vi "S4GUI.vi"(7 "Tab ObsEng":enum32{"Obs", "CCD modes", "Guider", "Eng"}(tab)) -> ()   [LabVIEW 2018] (continued)
        n5074 = call-dynamic "Write Focus.vi"("error in (no error)"=w12180, "GSdevice.lvclass"=w12182, "GSserver in"=w12181) -> ("error out"=w12177:errorcluster, "GSserver out"=w12179:refnum<class "GSserver.lvclass">)  [unwired: 7 in]
        n5075 = call-dynamic "Write GSserver.lvclass.vi"("error in (no error)"=w12177, "GSserver.lvclass"=w12179, "S4GUI in"=w12178) -> ("error out"=w12176:errorcluster, "S4GUI out"=w12175:refnum<class "S4GUI.lvclass">)  [unwired: 7 in]
      }
      event "GFOC_set": Value Change {
        n5076 = event-data() -> ()  [unwired: 1 in, 4 out]
        n5077 = call "Read Instrument.lvclass.vi"("error in (no error)"=w12207, "S4ACS_GUI in"=w12208) -> ("error out"=w12205:errorcluster, "Instrument.lvclass"=w12206:refnum<class "Instrument.lvclass">, "S4ACS_GUI out"=w12193:refnum<class "S4GUI.lvclass">)  [unwired: 7 in]
        n5078 = call "Read GFOC.vi"("error in (no error)"=w12205, "Instrument in"=w12206) -> ("error out"=w12202:errorcluster, "Opt_Continuous.lvclass"=w12204:refnum<class "Opt_Continuous.lvclass">, "Instrument out"=w12196:refnum<class "Instrument.lvclass">)  [unwired: 7 in]
        n5079 = call-dynamic "Read State Machine.vi"("error in (no error)"=w12202, "Device in"=w12204) -> ("error out"=w12201:errorcluster, "State Machine.lvclass"=w12190:refnum<class "State Machine.lvclass">, "Device out"=w12198:refnum<class "Opt_Continuous.lvclass">)  [unwired: 7 in]
        n5080 = call "Next State.vi"("error in (no error)"=w12201, "New_State"=1, "State Machine in"=w12190) -> ("error out"=w12200:errorcluster, "State Machine out"=w12199:refnum<class "State Machine.lvclass">)  [unwired: 7 in]
        n5081 = call-dynamic "Write State Machine.vi"("error in (no error)"=w12200, "State Machine.lvclass"=w12199, "Device in"=w12198) -> ("error out"=w12195:errorcluster, "Device out"=w12197:refnum<class "Opt_Continuous.lvclass">)  [unwired: 7 in]
        n5082 = call "Write GFOC.vi"("error in (no error)"=w12195, "Opt_Continuous.lvclass"=w12197, "Instrument in"=w12196) -> ("error out"=w12192:errorcluster, "Instrument out"=w12194:refnum<class "Instrument.lvclass">)  [unwired: 7 in]
        n5083 = call "Write Instrument.lvclass.vi"("error in (no error)"=w12192, "Instrument.lvclass"=w12194, "S4ACS_GUI in"=w12193) -> ("error out"=w12191:errorcluster, "S4ACS_GUI out"=w12189:refnum<class "S4GUI.lvclass">)  [unwired: 7 in]
      }
      event "GFOC_set 2": Value Change {
        n5084 = event-data() -> ()  [unwired: 1 in, 4 out]
        n5085 = call-dynamic "Read GSserver.lvclass.vi"("error in (no error)"=w12227, "S4GUI in"=w12228) -> ("error out"=w12225:errorcluster, "GSserver.lvclass"=w12226:refnum<class "GSserver.lvclass">, "S4GUI out"=w12213:refnum<class "S4GUI.lvclass">)  [unwired: 7 in]
        n5086 = call-dynamic "Read Focus.vi"("error in (no error)"=w12225, "GSserver in"=w12226) -> ("error out"=w12222:errorcluster, "GSdevice.lvclass"=w12224:refnum<class "GSdevice.lvclass">, "GSserver out"=w12216:refnum<class "GSserver.lvclass">)  [unwired: 7 in]
        n5087 = call-dynamic "Read State Machine.vi"("error in (no error)"=w12222, "Device in"=w12224) -> ("error out"=w12221:errorcluster, "State Machine.lvclass"=w12210:refnum<class "State Machine.lvclass">, "Device out"=w12218:refnum<class "GSdevice.lvclass">)  [unwired: 7 in]
        n5088 = call "Next State.vi"("error in (no error)"=w12221, "New_State"=10, "State Machine in"=w12210) -> ("error out"=w12220:errorcluster, "State Machine out"=w12219:refnum<class "State Machine.lvclass">)  [unwired: 7 in]
        n5089 = call-dynamic "Write State Machine.vi"("error in (no error)"=w12220, "State Machine.lvclass"=w12219, "Device in"=w12218) -> ("error out"=w12215:errorcluster, "Device out"=w12217:refnum<class "GSdevice.lvclass">)  [unwired: 7 in]
        n5090 = call-dynamic "Write Focus.vi"("error in (no error)"=w12215, "GSdevice.lvclass"=w12217, "GSserver in"=w12216) -> ("error out"=w12212:errorcluster, "GSserver out"=w12214:refnum<class "GSserver.lvclass">)  [unwired: 7 in]
        n5091 = call-dynamic "Write GSserver.lvclass.vi"("error in (no error)"=w12212, "GSserver.lvclass"=w12214, "S4GUI in"=w12213) -> ("error out"=w12211:errorcluster, "S4GUI out"=w12209:refnum<class "S4GUI.lvclass">)  [unwired: 7 in]
      }
      event "GFOC_stop", "GFOC_stop 2": Value Change {
        n5092 = event-data() -> ()  [unwired: 1 in, 4 out]
        n5093 = call "Read Instrument.lvclass.vi"("error in (no error)"=w12247, "S4ACS_GUI in"=w12248) -> ("error out"=w12245:errorcluster, "Instrument.lvclass"=w12246:refnum<class "Instrument.lvclass">, "S4ACS_GUI out"=w12232:refnum<class "S4GUI.lvclass">)  [unwired: 7 in]
        n5094 = call "Read GFOC.vi"("error in (no error)"=w12245, "Instrument in"=w12246) -> ("error out"=w12241:errorcluster, "Opt_Continuous.lvclass"=w12244:refnum<class "Opt_Continuous.lvclass">, "Instrument out"=w12235:refnum<class "Instrument.lvclass">)  [unwired: 7 in]
        n5095 = call-dynamic "Read State Machine.vi"("error in (no error)"=w12241, "Device in"=w12244) -> ("error out"=w12240:errorcluster, "State Machine.lvclass"=w12243:refnum<class "State Machine.lvclass">, "Device out"=w12237:refnum<class "Opt_Continuous.lvclass">)  [unwired: 7 in]
        n5096 = call "Next State.vi"("error in (no error)"=w12240, "New_State"=10, "State Machine in"=w12243) -> ("error out"=w12239:errorcluster, "State Machine out"=w12238:refnum<class "State Machine.lvclass">)  [unwired: 7 in]
        n5097 = call-dynamic "Write State Machine.vi"("error in (no error)"=w12239, "State Machine.lvclass"=w12238, "Device in"=w12237) -> ("error out"=w12234:errorcluster, "Device out"=w12236:refnum<class "Opt_Continuous.lvclass">)  [unwired: 7 in]
        n5098 = call "Write GFOC.vi"("error in (no error)"=w12234, "Opt_Continuous.lvclass"=w12236, "Instrument in"=w12235) -> ("error out"=w12231:errorcluster, "Instrument out"=w12233:refnum<class "Instrument.lvclass">)  [unwired: 7 in]
        n5099 = call "Write Instrument.lvclass.vi"("error in (no error)"=w12231, "Instrument.lvclass"=w12233, "S4ACS_GUI in"=w12232) -> ("error out"=w12230:errorcluster, "S4ACS_GUI out"=w12229:refnum<class "S4GUI.lvclass">)  [unwired: 7 in]
      }
      event "GFOC_init": Value Change {
        n5100 = event-data() -> ()  [unwired: 1 in, 4 out]
        n5101 = call "Read Instrument.lvclass.vi"("error in (no error)"=w12267, "S4ACS_GUI in"=w12268) -> ("error out"=w12265:errorcluster, "Instrument.lvclass"=w12266:refnum<class "Instrument.lvclass">, "S4ACS_GUI out"=w12252:refnum<class "S4GUI.lvclass">)  [unwired: 7 in]
        n5102 = call "Read GFOC.vi"("error in (no error)"=w12265, "Instrument in"=w12266) -> ("error out"=w12261:errorcluster, "Opt_Continuous.lvclass"=w12264:refnum<class "Opt_Continuous.lvclass">, "Instrument out"=w12255:refnum<class "Instrument.lvclass">)  [unwired: 7 in]
        n5103 = call-dynamic "Read State Machine.vi"("error in (no error)"=w12261, "Device in"=w12264) -> ("error out"=w12260:errorcluster, "State Machine.lvclass"=w12263:refnum<class "State Machine.lvclass">, "Device out"=w12257:refnum<class "Opt_Continuous.lvclass">)  [unwired: 7 in]
        n5104 = call "Next State.vi"("error in (no error)"=w12260, "New_State"=30, "State Machine in"=w12263) -> ("error out"=w12259:errorcluster, "State Machine out"=w12258:refnum<class "State Machine.lvclass">)  [unwired: 7 in]
        n5105 = call-dynamic "Write State Machine.vi"("error in (no error)"=w12259, "State Machine.lvclass"=w12258, "Device in"=w12257) -> ("error out"=w12254:errorcluster, "Device out"=w12256:refnum<class "Opt_Continuous.lvclass">)  [unwired: 7 in]
        n5106 = call "Write GFOC.vi"("error in (no error)"=w12254, "Opt_Continuous.lvclass"=w12256, "Instrument in"=w12255) -> ("error out"=w12251:errorcluster, "Instrument out"=w12253:refnum<class "Instrument.lvclass">)  [unwired: 7 in]
        n5107 = call "Write Instrument.lvclass.vi"("error in (no error)"=w12251, "Instrument.lvclass"=w12253, "S4ACS_GUI in"=w12252) -> ("error out"=w12250:errorcluster, "S4ACS_GUI out"=w12249:refnum<class "S4GUI.lvclass">)  [unwired: 7 in]
      }
      event "CALW_target": Value Change {
        n5108 = event-data() -> ("NewVal"=w12278:dbl)  [unwired: 1 in, 3 out]
        n5109 = call "Read Instrument.lvclass.vi"("error in (no error)"=w12282, "S4ACS_GUI in"=w12283) -> ("error out"=w12280:errorcluster, "Instrument.lvclass"=w12281:refnum<class "Instrument.lvclass">, "S4ACS_GUI out"=w12272:refnum<class "S4GUI.lvclass">)  [unwired: 7 in]
        n5110 = call "Read CALW.vi"("error in (no error)"=w12280, "Instrument in"=w12281) -> ("error out"=w12277:errorcluster, "Opt_Selector.lvclass"=w12279:refnum<class "Opt_Selector.lvclass">, "Instrument out"=w12275:refnum<class "Instrument.lvclass">)  [unwired: 7 in]
        n5111 = call "Write target.vi"("error in (no error)"=w12277, "target"=w12278, "Optics in"=w12279) -> ("error out"=w12274:errorcluster, "Optics out"=w12276:refnum<class "Opt_Selector.lvclass">)  [unwired: 7 in]
        n5112 = call "Write CALW.vi"("error in (no error)"=w12274, "Opt_Selector.lvclass"=w12276, "Instrument in"=w12275) -> ("error out"=w12271:errorcluster, "Instrument out"=w12273:refnum<class "Instrument.lvclass">)  [unwired: 7 in]
        n5113 = call "Write Instrument.lvclass.vi"("error in (no error)"=w12271, "Instrument.lvclass"=w12273, "S4ACS_GUI in"=w12272) -> ("error out"=w12270:errorcluster, "S4ACS_GUI out"=w12269:refnum<class "S4GUI.lvclass">)  [unwired: 7 in]
      }
      event "CALW_set": Value Change {
        n5114 = event-data() -> ()  [unwired: 1 in, 4 out]
        n5115 = call "Read Instrument.lvclass.vi"("error in (no error)"=w12302, "S4ACS_GUI in"=w12303) -> ("error out"=w12300:errorcluster, "Instrument.lvclass"=w12301:refnum<class "Instrument.lvclass">, "S4ACS_GUI out"=w12288:refnum<class "S4GUI.lvclass">)  [unwired: 7 in]
        n5116 = call "Read CALW.vi"("error in (no error)"=w12300, "Instrument in"=w12301) -> ("error out"=w12297:errorcluster, "Opt_Selector.lvclass"=w12299:refnum<class "Opt_Selector.lvclass">, "Instrument out"=w12291:refnum<class "Instrument.lvclass">)  [unwired: 7 in]
        n5117 = call-dynamic "Read State Machine.vi"("error in (no error)"=w12297, "Device in"=w12299) -> ("error out"=w12296:errorcluster, "State Machine.lvclass"=w12285:refnum<class "State Machine.lvclass">, "Device out"=w12293:refnum<class "Opt_Selector.lvclass">)  [unwired: 7 in]
        n5118 = call "Next State.vi"("error in (no error)"=w12296, "New_State"=1, "State Machine in"=w12285) -> ("error out"=w12295:errorcluster, "State Machine out"=w12294:refnum<class "State Machine.lvclass">)  [unwired: 7 in]
        n5119 = call-dynamic "Write State Machine.vi"("error in (no error)"=w12295, "State Machine.lvclass"=w12294, "Device in"=w12293) -> ("error out"=w12290:errorcluster, "Device out"=w12292:refnum<class "Opt_Selector.lvclass">)  [unwired: 7 in]
        n5120 = call "Write CALW.vi"("error in (no error)"=w12290, "Opt_Selector.lvclass"=w12292, "Instrument in"=w12291) -> ("error out"=w12287:errorcluster, "Instrument out"=w12289:refnum<class "Instrument.lvclass">)  [unwired: 7 in]
        n5121 = call "Write Instrument.lvclass.vi"("error in (no error)"=w12287, "Instrument.lvclass"=w12289, "S4ACS_GUI in"=w12288) -> ("error out"=w12286:errorcluster, "S4ACS_GUI out"=w12284:refnum<class "S4GUI.lvclass">)  [unwired: 7 in]
      }
      event "CALW_stop": Value Change {
        n5122 = event-data() -> ()  [unwired: 1 in, 4 out]
        n5123 = call "Read Instrument.lvclass.vi"("error in (no error)"=w12322, "S4ACS_GUI in"=w12323) -> ("error out"=w12320:errorcluster, "Instrument.lvclass"=w12321:refnum<class "Instrument.lvclass">, "S4ACS_GUI out"=w12307:refnum<class "S4GUI.lvclass">)  [unwired: 7 in]
        n5124 = call "Read CALW.vi"("error in (no error)"=w12320, "Instrument in"=w12321) -> ("error out"=w12316:errorcluster, "Opt_Selector.lvclass"=w12319:refnum<class "Opt_Selector.lvclass">, "Instrument out"=w12310:refnum<class "Instrument.lvclass">)  [unwired: 7 in]
        n5125 = call-dynamic "Read State Machine.vi"("error in (no error)"=w12316, "Device in"=w12319) -> ("error out"=w12315:errorcluster, "State Machine.lvclass"=w12318:refnum<class "State Machine.lvclass">, "Device out"=w12312:refnum<class "Opt_Selector.lvclass">)  [unwired: 7 in]
        n5126 = call "Next State.vi"("error in (no error)"=w12315, "New_State"=10, "State Machine in"=w12318) -> ("error out"=w12314:errorcluster, "State Machine out"=w12313:refnum<class "State Machine.lvclass">)  [unwired: 7 in]
        n5127 = call-dynamic "Write State Machine.vi"("error in (no error)"=w12314, "State Machine.lvclass"=w12313, "Device in"=w12312) -> ("error out"=w12309:errorcluster, "Device out"=w12311:refnum<class "Opt_Selector.lvclass">)  [unwired: 7 in]
        n5128 = call "Write CALW.vi"("error in (no error)"=w12309, "Opt_Selector.lvclass"=w12311, "Instrument in"=w12310) -> ("error out"=w12306:errorcluster, "Instrument out"=w12308:refnum<class "Instrument.lvclass">)  [unwired: 7 in]
        n5129 = call "Write Instrument.lvclass.vi"("error in (no error)"=w12306, "Instrument.lvclass"=w12308, "S4ACS_GUI in"=w12307) -> ("error out"=w12305:errorcluster, "S4ACS_GUI out"=w12304:refnum<class "S4GUI.lvclass">)  [unwired: 7 in]
      }
      event "CALW_init": Value Change {
        n5130 = event-data() -> ()  [unwired: 1 in, 4 out]
        n5131 = call "Read Instrument.lvclass.vi"("error in (no error)"=w12342, "S4ACS_GUI in"=w12343) -> ("error out"=w12340:errorcluster, "Instrument.lvclass"=w12341:refnum<class "Instrument.lvclass">, "S4ACS_GUI out"=w12327:refnum<class "S4GUI.lvclass">)  [unwired: 7 in]
        n5132 = call "Read CALW.vi"("error in (no error)"=w12340, "Instrument in"=w12341) -> ("error out"=w12336:errorcluster, "Opt_Selector.lvclass"=w12339:refnum<class "Opt_Selector.lvclass">, "Instrument out"=w12330:refnum<class "Instrument.lvclass">)  [unwired: 7 in]
        n5133 = call-dynamic "Read State Machine.vi"("error in (no error)"=w12336, "Device in"=w12339) -> ("error out"=w12335:errorcluster, "State Machine.lvclass"=w12338:refnum<class "State Machine.lvclass">, "Device out"=w12332:refnum<class "Opt_Selector.lvclass">)  [unwired: 7 in]
        n5134 = call "Next State.vi"("error in (no error)"=w12335, "New_State"=30, "State Machine in"=w12338) -> ("error out"=w12334:errorcluster, "State Machine out"=w12333:refnum<class "State Machine.lvclass">)  [unwired: 7 in]
        n5135 = call-dynamic "Write State Machine.vi"("error in (no error)"=w12334, "State Machine.lvclass"=w12333, "Device in"=w12332) -> ("error out"=w12329:errorcluster, "Device out"=w12331:refnum<class "Opt_Selector.lvclass">)  [unwired: 7 in]
        n5136 = call "Write CALW.vi"("error in (no error)"=w12329, "Opt_Selector.lvclass"=w12331, "Instrument in"=w12330) -> ("error out"=w12326:errorcluster, "Instrument out"=w12328:refnum<class "Instrument.lvclass">)  [unwired: 7 in]
        n5137 = call "Write Instrument.lvclass.vi"("error in (no error)"=w12326, "Instrument.lvclass"=w12328, "S4ACS_GUI in"=w12327) -> ("error out"=w12325:errorcluster, "S4ACS_GUI out"=w12324:refnum<class "S4GUI.lvclass">)  [unwired: 7 in]
      }
      event "ASEL_target": Value Change {
        n5138 = event-data() -> ("NewVal"=w12353:dbl)  [unwired: 1 in, 3 out]
        n5139 = call "Read Instrument.lvclass.vi"("error in (no error)"=w12357, "S4ACS_GUI in"=w12358) -> ("error out"=w12355:errorcluster, "Instrument.lvclass"=w12356:refnum<class "Instrument.lvclass">, "S4ACS_GUI out"=w12347:refnum<class "S4GUI.lvclass">)  [unwired: 7 in]
        n5140 = call "Read ASEL.vi"("error in (no error)"=w12355, "Instrument in"=w12356) -> ("error out"=w12352:errorcluster, "Opt_Selector.lvclass"=w12354:refnum<class "Opt_Selector.lvclass">, "Instrument out"=w12350:refnum<class "Instrument.lvclass">)  [unwired: 7 in]
        n5141 = call "Write target.vi"("error in (no error)"=w12352, "target"=w12353, "Optics in"=w12354) -> ("error out"=w12349:errorcluster, "Optics out"=w12351:refnum<class "Opt_Selector.lvclass">)  [unwired: 7 in]
        n5142 = call "Write ASEL.vi"("error in (no error)"=w12349, "Opt_Selector.lvclass"=w12351, "Instrument in"=w12350) -> ("error out"=w12346:errorcluster, "Instrument out"=w12348:refnum<class "Instrument.lvclass">)  [unwired: 7 in]
        n5143 = call "Write Instrument.lvclass.vi"("error in (no error)"=w12346, "Instrument.lvclass"=w12348, "S4ACS_GUI in"=w12347) -> ("error out"=w12345:errorcluster, "S4ACS_GUI out"=w12344:refnum<class "S4GUI.lvclass">)  [unwired: 7 in]
      }
      event "ASEL_set": Value Change {
        n5144 = event-data() -> ()  [unwired: 1 in, 4 out]
        n5145 = call "Read Instrument.lvclass.vi"("error in (no error)"=w12377, "S4ACS_GUI in"=w12378) -> ("error out"=w12375:errorcluster, "Instrument.lvclass"=w12376:refnum<class "Instrument.lvclass">, "S4ACS_GUI out"=w12363:refnum<class "S4GUI.lvclass">)  [unwired: 7 in]
        n5146 = call "Read ASEL.vi"("error in (no error)"=w12375, "Instrument in"=w12376) -> ("error out"=w12372:errorcluster, "Opt_Selector.lvclass"=w12374:refnum<class "Opt_Selector.lvclass">, "Instrument out"=w12366:refnum<class "Instrument.lvclass">)  [unwired: 7 in]
        n5147 = call-dynamic "Read State Machine.vi"("error in (no error)"=w12372, "Device in"=w12374) -> ("error out"=w12371:errorcluster, "State Machine.lvclass"=w12360:refnum<class "State Machine.lvclass">, "Device out"=w12368:refnum<class "Opt_Selector.lvclass">)  [unwired: 7 in]
        n5148 = call "Next State.vi"("error in (no error)"=w12371, "New_State"=1, "State Machine in"=w12360) -> ("error out"=w12370:errorcluster, "State Machine out"=w12369:refnum<class "State Machine.lvclass">)  [unwired: 7 in]
        n5149 = call-dynamic "Write State Machine.vi"("error in (no error)"=w12370, "State Machine.lvclass"=w12369, "Device in"=w12368) -> ("error out"=w12365:errorcluster, "Device out"=w12367:refnum<class "Opt_Selector.lvclass">)  [unwired: 7 in]
        n5150 = call "Write ASEL.vi"("error in (no error)"=w12365, "Opt_Selector.lvclass"=w12367, "Instrument in"=w12366) -> ("error out"=w12362:errorcluster, "Instrument out"=w12364:refnum<class "Instrument.lvclass">)  [unwired: 7 in]
        n5151 = call "Write Instrument.lvclass.vi"("error in (no error)"=w12362, "Instrument.lvclass"=w12364, "S4ACS_GUI in"=w12363) -> ("error out"=w12361:errorcluster, "S4ACS_GUI out"=w12359:refnum<class "S4GUI.lvclass">)  [unwired: 7 in]
      }
      event "ASEL_stop": Value Change {
        n5152 = event-data() -> ()  [unwired: 1 in, 4 out]
        n5153 = call "Read Instrument.lvclass.vi"("error in (no error)"=w12397, "S4ACS_GUI in"=w12398) -> ("error out"=w12395:errorcluster, "Instrument.lvclass"=w12396:refnum<class "Instrument.lvclass">, "S4ACS_GUI out"=w12382:refnum<class "S4GUI.lvclass">)  [unwired: 7 in]
        n5154 = call "Read ASEL.vi"("error in (no error)"=w12395, "Instrument in"=w12396) -> ("error out"=w12391:errorcluster, "Opt_Selector.lvclass"=w12394:refnum<class "Opt_Selector.lvclass">, "Instrument out"=w12385:refnum<class "Instrument.lvclass">)  [unwired: 7 in]
        n5155 = call-dynamic "Read State Machine.vi"("error in (no error)"=w12391, "Device in"=w12394) -> ("error out"=w12390:errorcluster, "State Machine.lvclass"=w12393:refnum<class "State Machine.lvclass">, "Device out"=w12387:refnum<class "Opt_Selector.lvclass">)  [unwired: 7 in]
        n5156 = call "Next State.vi"("error in (no error)"=w12390, "New_State"=10, "State Machine in"=w12393) -> ("error out"=w12389:errorcluster, "State Machine out"=w12388:refnum<class "State Machine.lvclass">)  [unwired: 7 in]
        n5157 = call-dynamic "Write State Machine.vi"("error in (no error)"=w12389, "State Machine.lvclass"=w12388, "Device in"=w12387) -> ("error out"=w12384:errorcluster, "Device out"=w12386:refnum<class "Opt_Selector.lvclass">)  [unwired: 7 in]
        n5158 = call "Write ASEL.vi"("error in (no error)"=w12384, "Opt_Selector.lvclass"=w12386, "Instrument in"=w12385) -> ("error out"=w12381:errorcluster, "Instrument out"=w12383:refnum<class "Instrument.lvclass">)  [unwired: 7 in]
        n5159 = call "Write Instrument.lvclass.vi"("error in (no error)"=w12381, "Instrument.lvclass"=w12383, "S4ACS_GUI in"=w12382) -> ("error out"=w12380:errorcluster, "S4ACS_GUI out"=w12379:refnum<class "S4GUI.lvclass">)  [unwired: 7 in]
      }
      event "ASEL_init": Value Change {
        n5160 = event-data() -> ()  [unwired: 1 in, 4 out]
        n5161 = call "Read Instrument.lvclass.vi"("error in (no error)"=w12417, "S4ACS_GUI in"=w12418) -> ("error out"=w12415:errorcluster, "Instrument.lvclass"=w12416:refnum<class "Instrument.lvclass">, "S4ACS_GUI out"=w12402:refnum<class "S4GUI.lvclass">)  [unwired: 7 in]
        n5162 = call "Read ASEL.vi"("error in (no error)"=w12415, "Instrument in"=w12416) -> ("error out"=w12411:errorcluster, "Opt_Selector.lvclass"=w12414:refnum<class "Opt_Selector.lvclass">, "Instrument out"=w12405:refnum<class "Instrument.lvclass">)  [unwired: 7 in]
        n5163 = call-dynamic "Read State Machine.vi"("error in (no error)"=w12411, "Device in"=w12414) -> ("error out"=w12410:errorcluster, "State Machine.lvclass"=w12413:refnum<class "State Machine.lvclass">, "Device out"=w12407:refnum<class "Opt_Selector.lvclass">)  [unwired: 7 in]
        n5164 = call "Next State.vi"("error in (no error)"=w12410, "New_State"=30, "State Machine in"=w12413) -> ("error out"=w12409:errorcluster, "State Machine out"=w12408:refnum<class "State Machine.lvclass">)  [unwired: 7 in]
        n5165 = call-dynamic "Write State Machine.vi"("error in (no error)"=w12409, "State Machine.lvclass"=w12408, "Device in"=w12407) -> ("error out"=w12404:errorcluster, "Device out"=w12406:refnum<class "Opt_Selector.lvclass">)  [unwired: 7 in]
        n5166 = call "Write ASEL.vi"("error in (no error)"=w12404, "Opt_Selector.lvclass"=w12406, "Instrument in"=w12405) -> ("error out"=w12401:errorcluster, "Instrument out"=w12403:refnum<class "Instrument.lvclass">)  [unwired: 7 in]
        n5167 = call "Write Instrument.lvclass.vi"("error in (no error)"=w12401, "Instrument.lvclass"=w12403, "S4ACS_GUI in"=w12402) -> ("error out"=w12400:errorcluster, "S4ACS_GUI out"=w12399:refnum<class "S4GUI.lvclass">)  [unwired: 7 in]
      }
    }
    n5168 = Unbundle By Name(w122) -> ("status"=w121:bool)
    n5169 = flat-sequence {
      tunnel: w136 -> [w151]
      tunnel: w134 -> [w149]
      tunnel: [w151] -> w133
      tunnel: [w147] -> w132
      tunnel: [w146] -> w131
      tunnel: [w154] -> w135
      tunnel: w133 -> [w154]
      tunnel: w132 -> [w153]
      tunnel: w131 -> [w152]
      frame #0 {
        n5170 = Tick Count (ms)() -> (millisecond timer value=w150:u32)
        n5171 = local read "loop max(ms)"() -> (w145:u32)
        n5172 = Subtract(x=w150, y=w149) -> (x-y=w147:u32)
        n5173 = Greater?(x=w147, y=w145) -> (0:w148:bool)
        n5174 = Select(t=w147, s=w148, f=w145) -> (s? t:f=w146:u32)
      }
      frame #1 {
        "loop time(ms)" <- w153
        "loop max(ms)" <- w152
      }
    }
    n5175 = Or(x=w121, y=w120) -> (x .or. y?=w119:bool)
  }
  "error out 9" <- w2
  n5176 = while {
    tunnel: w9 -> [_]
    stop <- FALSE stop-if-true
    n5177 = disable-structure shown="Enabled" {
      frame Disabled {
        n5178 = call "ZeroMQ_ACS1.vi"() -> ()  [unwired: 12 in]
        n5179 = call "ZeroMQ_ACS2.vi"() -> ()  [unwired: 12 in]
        n5180 = call "ZeroMQ_ACS3.vi"() -> ()  [unwired: 12 in]
        n5181 = call "ZeroMQ_ACS4.vi"() -> ()  [unwired: 12 in]
        n5182 = disable-structure shown="Enabled" {
          frame Disabled {
            n5183 = call "ZeroMQ_FOC.vi"() -> ()  [unwired: 12 in]
          }
          frame Enabled {
            n5184 = call "ZeroMQ_FOC_REQREP.vi"() -> ()  [unwired: 12 in]
          }
        }
        n5185 = call "ZeroMQ_WSTA.vi"() -> ()  [unwired: 12 in]
        n5186 = call "ZeroMQ_TCS.vi"() -> ()  [unwired: 12 in]
        n5187 = call "ZeroMQ_S4ICS.vi"() -> ()  [unwired: 12 in]
        n5188 = call "ZeroMQ_SUBGS.vi"() -> ()  [unwired: 12 in]
        n5189 = call "StreamTransmitSyncBox.vi"() -> ()  [unwired: 12 in]
        n5190 = call "StreamReceiveSyncBox.vi"() -> ()  [unwired: 12 in]
        n5191 = call "ZeroMQ_PUB.vi"() -> ()  [unwired: 12 in]
      }
      frame Enabled {
        n5192 = call "communication manager.vi"() -> ()  [unwired: 12 in]
      }
    }
  }
  n5193 = stacked-sequence "INTERFACE" {
    frame #0 {
    }
    frame #1 {
    }
    frame #2 {
    }
    frame #3 {
    }
    frame #4 {
    }
  }
  n5194 = call-dynamic "Log Error.vi"("error in (no error)"=w2, "S4GUI in"=w4) -> ("error out"=→"error out 10":errorcluster, "S4GUI out"=w3:refnum<class "S4GUI.lvclass">)  [unwired: 8 in]
  n5195 = call-dynamic "End.vi"("S4ACS_GUI in"=w3) -> ("error out"=w21:errorcluster)  [unwired: 9 in, 1 out]
  n5196 = flat-sequence {
    tunnel: [w12421] -> w19
    tunnel: w21 -> [w12423]
    tunnel: [w12429] -> w20
    tunnel: w19 -> [w12429]
    frame #0 {
      w12427 = FALSE
      # "Apaga todos os leds, habilita Tab ObsEng."
      n5197 = property on="Tab ObsEng" class="TabCtl (strict)"("Tabs Visible?"=TRUE) -> ()  [unwired: 2 in, 2 out]
      n5198 = property on="Channel 4" class="Bool (strict)"("Value"=w12427) -> ()  [unwired: 2 in, 2 out]
      n5199 = property on="Channel 3" class="Bool (strict)"("Value"=w12427) -> ()  [unwired: 2 in, 2 out]
      n5200 = property on="Channel 2" class="Bool (strict)"("Value"=w12427) -> ()  [unwired: 2 in, 2 out]
      n5201 = property on="Channel 1" class="Bool (strict)"("Value"=w12427) -> ()  [unwired: 2 in, 2 out]
      n5202 = property on="S4ICSoft" class="Bool (strict)"("Value"=w12427) -> ()  [unwired: 2 in, 2 out]
      n5203 = call <vilib>:"Clear Errors.vi"("error in (no error)"=w12423) -> ("error out"=w12420:errorcluster)  [unwired: 5 in, 1 out]
      n5204 = property on="TCSPD" class="Bool (strict)"("Value"=w12427) -> ()  [unwired: 2 in, 2 out]
      n5205 = property on="Focus 160" class="Bool (strict)"("Value"=w12427) -> ()  [unwired: 2 in, 2 out]
      n5206 = property on="Weather" class="Bool (strict)"("Value"=w12427) -> ()  [unwired: 2 in, 2 out]
      n5207 = property on="GUIDER" class="Bool (strict)"("Value"=w12427) -> ()  [unwired: 2 in, 2 out]
      n5208 = disable-structure shown="Disabled" {
        frame Disabled {
          n5209 = local write "Last Error"("" ("Last Error")) -> ()
        }
        frame Enabled {
        }
      }
      n5210 = property on="Last Error" class="Str"(error in=w12420, "Text.BG Color"=u32 13816530 ("Color Box"), "Caption.FontBold"=FALSE ("Caption.Font:Bold")) -> (error out=w12422:errorcluster)  [unwired: 1 in, 1 out]
      n5211 = call <vilib>:"Clear Errors.vi"("error in (no error)"=w12422) -> ("error out"=w12421:errorcluster)  [unwired: 5 in, 1 out]
    }
    frame #1 {
      n5212 = Stop() -> ()  [unwired: 1 in]
    }
  }
  "error out" <- w20
  "GUI version" <- w22
